vi "pupila_object_tracking_VI_1.vi"() -> ()   [LabVIEW 2024]
doc: "Este VI realiza la detección de la pupila de un ojo humano, y mediante el uso de Vision Assistant procesa la imagen para realizar un seguimiento de la pupila, así como regresa información de la posición del objeto, y con esto se acciona una entrada de teclado. \n\nAutores:\nIvan Nieto Guerrero, David Alejandro Zarazúa Martínez.\n\n06/May/2025"
uses:
  <vilib>/userDefined/High Color/IMAQdx.ctl
  <vilib>/vision/driver/NI_Vision_Acquisition_Software.lvlib
panel:
  in  "Texto":string
  out "Datos de poisición":T1(array[cluster])
  in  "left":bool
  in  "right":bool
  in  "top":bool
  in  "down":bool
  out "Posición":cluster{"X":dbl, "Y":dbl}[](graph)
  in  "stop":bool
  out "Cámara":T2(plugin-control)
  # "Detección de la pupila"
  # "Este programa adquiere la posición de la pupila y de acuerdo en donde se posicione podrá accionar una letra del teclado de manera automática."
  # "Mire hacia la pantalla, NO MIRAR DIRECTAMENTE A LA CÁMARA.\nColoque el ojo en el centro del recuadro, procurando que la pupila quede en el centro de la cruz verde."
  # "Datos de la pupila."
  # "La gráfica muestra la posición de la pupila respecto a la cruz."
  # "Controles que muestran la orientación de la pupila respecto a la cruz verde."
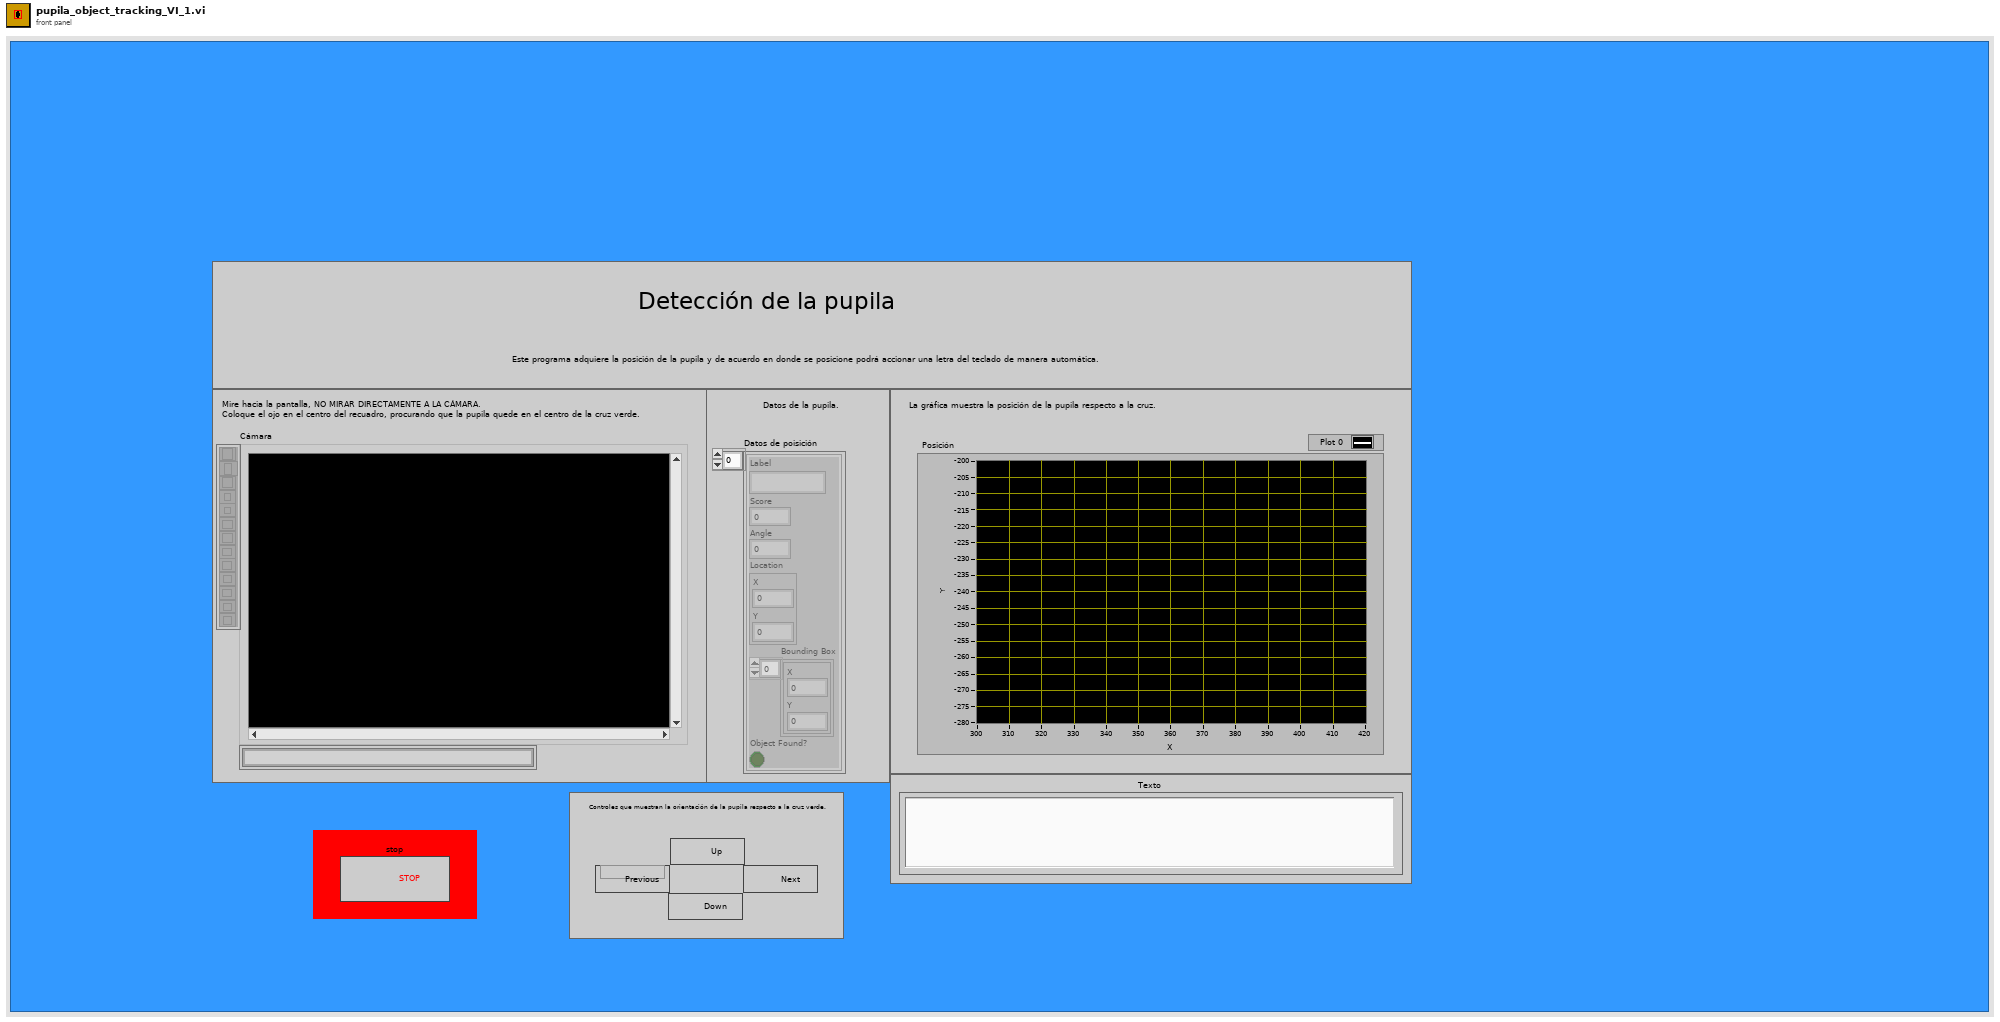
[diagram p1: front panel]
types:
  T1 = cluster{"Label":string, "Score":i32, "Angle":dbl, "Location":cluster{"X":dbl, "Y":dbl}, "Bounding Box":cluster{"X":dbl, "Y":dbl}[], "Object Found?":bool}[]
  T2 = typedef "IMAQ Image.ctl" = refnum<image>
  T3 = typedef "IMAQdx.ctl" = refnum<k21>
  T4 = cluster{"Label":string, "Score":i32, "Angle":dbl, "Location":cluster{"X":dbl, "Y":dbl}, "Bounding Box":cluster{"X":dbl, "Y":dbl}[], "Object Found?":bool}
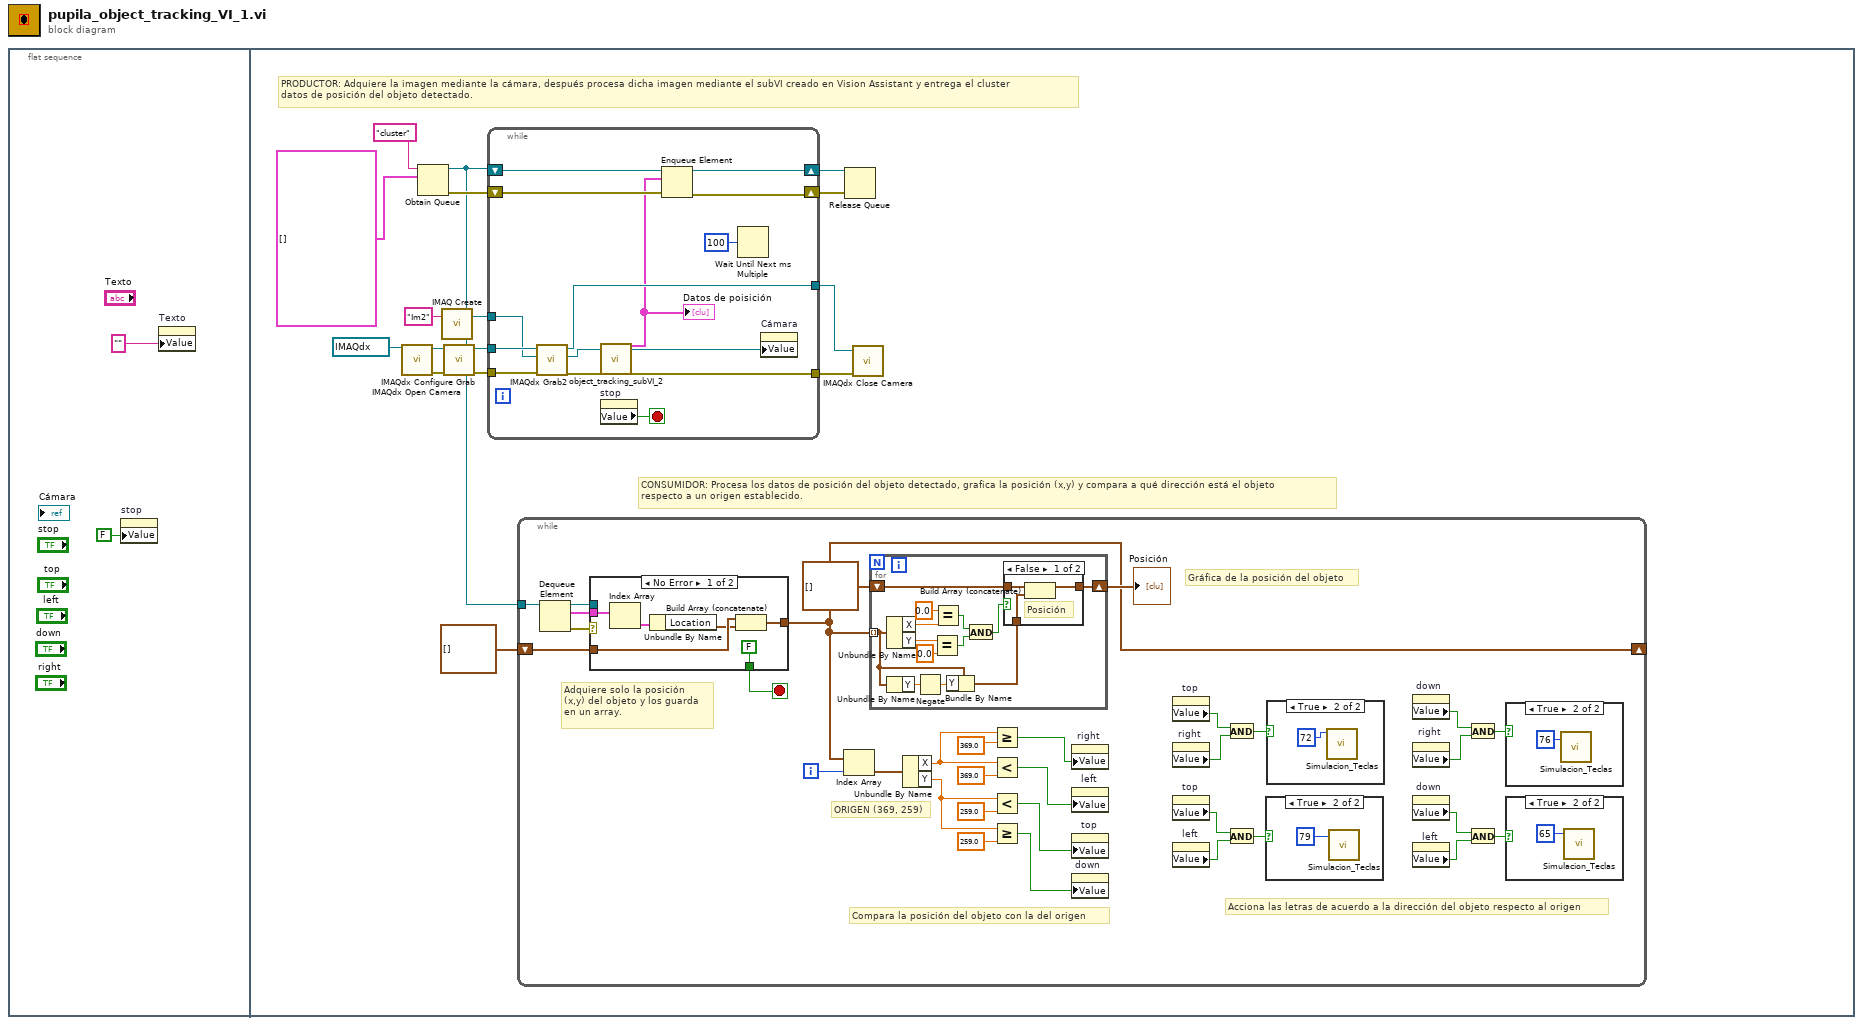
[diagram p0: block diagram]
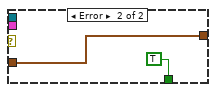
[diagram p7: hidden frame]
diagram:
  n1 = flat-sequence {
    frame #0 {
      n2 = property on="stop" class="Bool (strict)"("Value"=FALSE ("stop")) -> ()  [unwired: 2 in, 2 out]
      n3 = property on="Texto" class="Str"("Value"="") -> ()  [unwired: 2 in, 2 out]
    }
    frame #1 {
      # "CONSUMIDOR: Procesa los datos de posición del objeto detectado, grafica la posición (x,y) y compara a qué dirección está el objeto\nrespecto a un origen establecido."
      # "PRODUCTOR: Adquiere la imagen mediante la cámara, después procesa dicha imagen mediante el subVI creado en Vision Assistant y entrega el cluster \ndatos de posición del objeto detectado."
      n4 = call <vilib>:"IMAQdx Open Camera.vi"("Session In"=T3 "cam1") -> ("error out"=w18:errorcluster, "Session Out"=w17:T3)  [unwired: 9 in]
      n5 = Obtain Queue(name (unnamed)="cluster", element data type=T1 [] ("Objects (pixel) (Object Tracking 1)")) -> (queue out=w7:refnum<queue>, error out=w8:errorcluster)  [unwired: 3 in, 1 out]
      n6 = call "IMAQ Create"("Image Name"="Im2") -> ("New Image"=w14:T2)  [unwired: 4 in, 1 out]
      n7 = call <vilib>:"IMAQdx Configure Grab.vi"("error in"=w18, "Session In"=w17) -> ("error out"=w12:errorcluster, "Session Out"=w13:T3)  [unwired: 8 in]
      n8 = while {
        tunnel: w14 -> [w94]
        tunnel: w13 -> [w95]
        tunnel: w12 -> [w93]
        tunnel: [w86] -> w11
        tunnel: [w82] -> w10
        shift-right: [w91] -> w4
        shift-left: w7 -> [w92]
        shift-right: [w89] -> w5
        shift-left: w8 -> [w90]
        stop <- w83 stop-if-true
        n9 = call <vilib>:"IMAQdx Grab2.vi"("error in"=w93, "Image In"=w94, "Session In"=w95) -> ("error out"=w87:errorcluster, "Image Out"=w85:T2, "Session Out"=w86:T3)  [unwired: 5 in, 1 out]
        n10 = call "object_tracking_subVI_2.vi"("Image"=w85, "error in"=w87) -> ("Objects (pixel) (Object Tracking 1)"=w84:T1, "Image Out"=w81:T2, "error out"=w82:errorcluster)  [unwired: 23 in]
        "Datos de poisición" <- w84
        n11 = property on="stop" class="Bool (strict)"() -> ("Value"=w83:bool)  [unwired: 2 in, 2 out]
        n12 = Enqueue Element(queue=w92, element=w84, error in (no error)=w90) -> (queue out=w91:refnum<queue>, error out=w89:errorcluster)  [unwired: 1 in, 1 out]
        n13 = Wait Until Next ms Multiple(millisecond multiple=u32 100) -> ()  [unwired: 1 out]
        n14 = property on="Cámara" class="ImageControl"("Value"=w81) -> ()  [unwired: 2 in, 2 out]
      }
      n15 = while {
        tunnel: w7 -> [w51]
        shift-right: [w33] -> _
        shift-left: cluster{"X":dbl, "Y":dbl}[] [] -> [w47]
        i -> [w32]
        stop <- w46 stop-if-true
        # "Acciona las letras de acuerdo a la dirección del objeto respecto al origen"
        # "Compara la posición del objeto con la del origen"
        # "ORIGEN (369, 259)"
        # "Adquiere solo la posición \n(x,y) del objeto y los guarda \nen un array."
        # "Gráfica de la posición del objeto"
        n16 = Dequeue Element(queue=w51) -> (queue out=w49:refnum<queue>, element=w48:T1, error out=w50:errorcluster)  [unwired: 2 in, 1 out]
        n17 = case shown="No Error" w50 {
          tunnel: w49 -> [_ _]
          tunnel: w48 -> [w78 _]
          tunnel: w47 -> [w76 w80]
          tunnel: [w74 w80] -> w33
          tunnel: [FALSE TRUE] -> w46
          frame No Error {
            n18 = Index Array(array=w78) -> (element=w77:T4)  [unwired: 1 in]
            n19 = Unbundle By Name(w77) -> ("Location"=w75:cluster{"X":dbl, "Y":dbl})
            n20 = Build Array (concatenate)(w76, w75) -> (w74:cluster{"X":dbl, "Y":dbl}[])
          }
          frame Error {
          }
        }
        n21 = Index Array(array=w33, index=w32) -> (element=w31:cluster{"X":dbl, "Y":dbl})
        n22 = for {
          tunnel: w33 -> [w60] mode=indexing
          shift-right: [w63] -> w44
          shift-left: cluster{"X":dbl, "Y":dbl}[] [] -> [w64]
          n23 = Unbundle By Name(w60) -> ("X"=w66:dbl, "Y"=w65:dbl)
          n24 = Unbundle By Name(w60) -> ("Y"=w62:dbl)
          n25 = Negate(x=w62) -> (-x=w61:dbl)
          n26 = Equal?(x=w65, y=0.0) -> (x = y?=w68:bool)
          n27 = Equal?(x=0.0, y=w66) -> (x = y?=w67:bool)
          n28 = Bundle By Name(cluster=w60, "Y"=w61) -> (w58:cluster{"X":dbl, "Y":dbl})
          n29 = And(x=w67, y=w68) -> (x .and. y?=w59:bool)
          n30 = case shown="False" w59 {
            tunnel: w64 -> [w69 w72]
            tunnel: [w71 w72] -> w63
            tunnel: w58 -> [w70 _]
            frame False {
              # "Posición"
              n31 = Build Array (concatenate)(w69, w70) -> (w71:cluster{"X":dbl, "Y":dbl}[])
            }
            frame True {
            }
          }
        }
        "Posición" <- w44
        n32 = Unbundle By Name(w31) -> ("X"=w41:dbl, "Y"=w39:dbl)
        n33 = Greater Or Equal?(x=w41, y=369.0) -> (x >= y?=w38:bool)
        n34 = Less?(x=w41, y=369.0) -> (x < y?=w37:bool)
        n35 = Less?(x=w39, y=259.0) -> (x < y?=w36:bool)
        n36 = Greater Or Equal?(x=w39, y=259.0) -> (x >= y?=w35:bool)
        n37 = property on="right" class="Bool (strict)"("Value"=w38) -> ()  [unwired: 2 in, 2 out]
        n38 = property on="left" class="Bool (strict)"("Value"=w37) -> ()  [unwired: 2 in, 2 out]
        n39 = property on="top" class="Bool (strict)"("Value"=w36) -> ()  [unwired: 2 in, 2 out]
        n40 = property on="down" class="Bool (strict)"("Value"=w35) -> ()  [unwired: 2 in, 2 out]
        n41 = property on="top" class="Bool (strict)"() -> ("Value"=w29:bool)  [unwired: 2 in, 2 out]
        n42 = property on="right" class="Bool (strict)"() -> ("Value"=w28:bool)  [unwired: 2 in, 2 out]
        n43 = property on="top" class="Bool (strict)"() -> ("Value"=w27:bool)  [unwired: 2 in, 2 out]
        n44 = property on="left" class="Bool (strict)"() -> ("Value"=w22:bool)  [unwired: 2 in, 2 out]
        n45 = And(x=w29, y=w28) -> (x .and. y?=w30:bool)
        n46 = And(x=w27, y=w22) -> (x .and. y?=w26:bool)
        n47 = case shown="True" w26 {
          frame False {
          }
          frame True {
            n48 = call "Simulacion_Teclas.vi"("Numeric"=79) -> ()  [unwired: 11 in]
          }
        }
        n49 = case shown="True" w30 {
          frame False {
          }
          frame True {
            n50 = call "Simulacion_Teclas.vi"("Numeric"=72) -> ()  [unwired: 11 in]
          }
        }
        n51 = property on="down" class="Bool (strict)"() -> ("Value"=w19:bool)  [unwired: 2 in, 2 out]
        n52 = property on="right" class="Bool (strict)"() -> ("Value"=w24:bool)  [unwired: 2 in, 2 out]
        n53 = property on="down" class="Bool (strict)"() -> ("Value"=w20:bool)  [unwired: 2 in, 2 out]
        n54 = property on="left" class="Bool (strict)"() -> ("Value"=w21:bool)  [unwired: 2 in, 2 out]
        n55 = And(x=w19, y=w24) -> (x .and. y?=w25:bool)
        n56 = And(x=w20, y=w21) -> (x .and. y?=w23:bool)
        n57 = case shown="True" w25 {
          frame False {
          }
          frame True {
            n58 = call "Simulacion_Teclas.vi"("Numeric"=76) -> ()  [unwired: 11 in]
          }
        }
        n59 = case shown="True" w23 {
          frame False {
          }
          frame True {
            n60 = call "Simulacion_Teclas.vi"("Numeric"=65) -> ()  [unwired: 11 in]
          }
        }
      }
      n61 = Release Queue(queue=w4, error in (no error)=w5) -> ()  [unwired: 1 in, 3 out]
      n62 = call <vilib>:"IMAQdx Close Camera.vi"("error in"=w10, "Session In"=w11) -> ()  [unwired: 9 in, 1 out]
    }
  }
